vi "输入数据解析.vi"(0 "单个参数补充":dbl, 1 "从板号":dbl=1.0, 2 "主板二维码":string="BNET01", 3 "从板二维码":string="BNET01", 5 "主板引用":refnum<vi>, 7 "从板引用":refnum<vi>, 9 "主板选项":string="三级故障阀值", 11 "枚举":enum16{"主板", "从板"}(ring), 12 "快换":bool caption="快换写入") -> (4 "输出数组":dbl[][](array[numeric]), 6 "数组长度":dbl[](array[numeric]), 8 "循环次数":i32, 10 "命令":u32, 14 "名称":string[](array[string]), 15 "命令序号":u32[](array[numeric]))   [LabVIEW 2013] (continued)
              tunnel: [w18491 w18502 w18513 w18524 w18534 w18544 w18555] -> w18485
              frame 0, Default {
                # "电压过高"
                n7255 = disable-structure shown="启用" {
                  disable-tunnel: [w18497 w18500] -> w18493
                  disable-tunnel: [w18496 w18500] -> w18492
                  disable-tunnel: w18490 -> [w18495 _]
                  frame Disabled {
                    n7256 = Unbundle By Name(w18495) -> ("电压过高"=w18494:dbl)
                    n7257 = call "输入分辨率计算-EV05.vi"("1字节?"=FALSE, "数值"=w18494, "分辨率"=0.1) -> ("低字节"=w18496:dbl, "高字节1"=w18497:dbl)  [unwired: 2 in, 5 out]
                  }
                  frame Enabled {
                    w18500 = 255 ("高字节1")
                  }
                }
                n7258 = Build Array(w18493, w18492) -> (w18491:i32[])
              }
              frame 1 {
                # "电压过低"
                n7259 = disable-structure shown="启用" {
                  disable-tunnel: [w18508 w18511] -> w18504
                  disable-tunnel: [w18507 w18511] -> w18503
                  disable-tunnel: w18501 -> [w18506 _]
                  frame Disabled {
                    n7260 = Unbundle By Name(w18506) -> ("电压过低"=w18505:dbl)
                    n7261 = call "输入分辨率计算-EV05.vi"("1字节?"=FALSE, "数值"=w18505, "分辨率"=0.1) -> ("低字节"=w18507:dbl, "高字节1"=w18508:dbl)  [unwired: 2 in, 5 out]
                  }
                  frame Enabled {
                    w18511 = 255 ("高字节1")
                  }
                }
                n7262 = Build Array(w18504, w18503) -> (w18502:i32[])
              }
              frame 2 {
                # "电压不均衡"
                n7263 = disable-structure shown="启用" {
                  disable-tunnel: [w18519 w18522] -> w18515
                  disable-tunnel: [w18518 w18522] -> w18514
                  disable-tunnel: w18512 -> [w18517 _]
                  frame Disabled {
                    n7264 = Unbundle By Name(w18517) -> ("电压不均衡(V)"=w18516:dbl)
                    n7265 = call "输入分辨率计算-EV05.vi"("1字节?"=FALSE, "数值"=w18516, "分辨率"=0.1) -> ("低字节"=w18518:dbl, "高字节1"=w18519:dbl)  [unwired: 2 in, 5 out]
                  }
                  frame Enabled {
                    w18522 = 255 ("高字节1")
                  }
                }
                n7266 = Build Array(w18515, w18514) -> (w18513:i32[])
              }
              frame 3 {
                # "温度过高"
                n7267 = disable-structure shown="启用" {
                  disable-tunnel: [w18529 255 ("高字节1")] -> w18525
                  disable-tunnel: w18523 -> [w18527 _]
                  frame Disabled {
                    n7268 = Unbundle By Name(w18527) -> ("温度过高"=w18526:dbl)
                    n7269 = call "输入分辨率计算-EV05.vi"("1字节?"=TRUE, "数值"=w18526, "偏移量"=-40.0, "分辨率"=1.0) -> ("高字节1"=w18529:dbl)  [unwired: 1 in, 6 out]
                  }
                  frame Enabled {
                  }
                }
                n7270 = Build Array(w18525) -> (w18524:i32[])
              }
              frame 4 {
                # "温度过低"
                n7271 = disable-structure shown="启用" {
                  disable-tunnel: [w18539 255 ("高字节1")] -> w18535
                  disable-tunnel: w18533 -> [w18537 _]
                  frame Disabled {
                    n7272 = Unbundle By Name(w18537) -> ("温度过低"=w18536:dbl)
                    n7273 = call "输入分辨率计算-EV05.vi"("1字节?"=TRUE, "数值"=w18536, "偏移量"=-40.0, "分辨率"=1.0) -> ("高字节1"=w18539:dbl)  [unwired: 1 in, 6 out]
                  }
                  frame Enabled {
                  }
                }
                n7274 = Build Array(w18535) -> (w18534:i32[])
              }
              frame 5 {
                # "温度不均衡"
                n7275 = disable-structure shown="启用" {
                  disable-tunnel: [w18548 255 ("高字节1")] -> w18545
                  disable-tunnel: w18543 -> [w18547 _]
                  frame Disabled {
                    n7276 = Unbundle By Name(w18547) -> ("温度不均衡"=w18546:dbl)
                    n7277 = call "输入分辨率计算-EV05.vi"("1字节?"=TRUE, "数值"=w18546, "分辨率"=1.0) -> ("高字节1"=w18548:dbl)  [unwired: 2 in, 6 out]
                  }
                  frame Enabled {
                  }
                }
                n7278 = Build Array(w18545) -> (w18544:i32[])
              }
              frame 6 {
                # "SOC过低"
                n7279 = disable-structure shown="启用" {
                  disable-tunnel: w18554 -> [w18559 _]
                  disable-tunnel: [w18556 w18562] -> w18553
                  disable-tunnel: [w18557 w18562] -> w18552
                  frame Enabled {
                    n7280 = Unbundle By Name(w18559) -> ("SOC过低"=w18558:dbl)
                    n7281 = call "输入分辨率计算-EV05.vi"("1字节?"=FALSE, "数值"=w18558, "分辨率"=0.1) -> ("低字节"=w18556:dbl, "高字节1"=w18557:dbl)  [unwired: 2 in, 5 out]
                  }
                  frame Disabled {
                    w18562 = 255 ("高字节1")
                  }
                }
                n7282 = Build Array(w18552, w18553) -> (w18555:dbl[])
              }
            }
            n7283 = Insert Into Array(array=w18486, new element=w18485) -> (w18487:dbl[])  [unwired: 1 in]
          }
          n7284 = Build Array(w18480) -> (w18479:dbl[][])
        }
        frame "SOC过低(2)" {
          n7285 = Unbundle By Name(w18567) -> ("二级故障(从板)"=w18568:refnum<vi>)
          n7286 = property class="Clust (严格)"(reference=w18568) -> ("Value"=w18566:T8)  [unwired: 1 in, 2 out]
          n7287 = for {
            N: 7 -> [_]
            tunnel: w18566 -> [w18578]
            shift-right: [w18577] -> w18570
            shift-left: dbl[] [] -> [w18576]
            i -> [w18579]
            n7288 = case shown="6" w18579 {
              tunnel: w18578 -> [w18580 w18591 w18602 w18613 w18623 w18633 w18644]
              tunnel: [w18581 w18592 w18603 w18614 w18624 w18634 w18645] -> w18575
              frame 0, Default {
                # "电压过高"
                n7289 = disable-structure shown="启用" {
                  disable-tunnel: [w18587 w18590] -> w18583
                  disable-tunnel: [w18586 w18590] -> w18582
                  disable-tunnel: w18580 -> [w18585 _]
                  frame Disabled {
                    n7290 = Unbundle By Name(w18585) -> ("电压过高"=w18584:dbl)
                    n7291 = call "输入分辨率计算-EV05.vi"("1字节?"=FALSE, "数值"=w18584, "分辨率"=0.1) -> ("低字节"=w18586:dbl, "高字节1"=w18587:dbl)  [unwired: 2 in, 5 out]
                  }
                  frame Enabled {
                    w18590 = 255 ("高字节1")
                  }
                }
                n7292 = Build Array(w18583, w18582) -> (w18581:i32[])
              }
              frame 1 {
                # "电压过低"
                n7293 = disable-structure shown="启用" {
                  disable-tunnel: [w18598 w18601] -> w18594
                  disable-tunnel: [w18597 w18601] -> w18593
                  disable-tunnel: w18591 -> [w18596 _]
                  frame Disabled {
                    n7294 = Unbundle By Name(w18596) -> ("电压过低"=w18595:dbl)
                    n7295 = call "输入分辨率计算-EV05.vi"("1字节?"=FALSE, "数值"=w18595, "分辨率"=0.1) -> ("低字节"=w18597:dbl, "高字节1"=w18598:dbl)  [unwired: 2 in, 5 out]
                  }
                  frame Enabled {
                    w18601 = 255 ("高字节1")
                  }
                }
                n7296 = Build Array(w18594, w18593) -> (w18592:i32[])
              }
              frame 2 {
                # "电压不均衡"
                n7297 = disable-structure shown="启用" {
                  disable-tunnel: [w18609 w18612] -> w18605
                  disable-tunnel: [w18608 w18612] -> w18604
                  disable-tunnel: w18602 -> [w18607 _]
                  frame Disabled {
                    n7298 = Unbundle By Name(w18607) -> ("电压不均衡(V)"=w18606:dbl)
                    n7299 = call "输入分辨率计算-EV05.vi"("1字节?"=FALSE, "数值"=w18606, "分辨率"=0.1) -> ("低字节"=w18608:dbl, "高字节1"=w18609:dbl)  [unwired: 2 in, 5 out]
                  }
                  frame Enabled {
                    w18612 = 255 ("高字节1")
                  }
                }
                n7300 = Build Array(w18605, w18604) -> (w18603:i32[])
              }
              frame 3 {
                # "温度过高"
                n7301 = disable-structure shown="启用" {
                  disable-tunnel: [w18619 255 ("高字节1")] -> w18615
                  disable-tunnel: w18613 -> [w18617 _]
                  frame Disabled {
                    n7302 = Unbundle By Name(w18617) -> ("温度过高"=w18616:dbl)
                    n7303 = call "输入分辨率计算-EV05.vi"("1字节?"=TRUE, "数值"=w18616, "偏移量"=-40.0, "分辨率"=1.0) -> ("高字节1"=w18619:dbl)  [unwired: 1 in, 6 out]
                  }
                  frame Enabled {
                  }
                }
                n7304 = Build Array(w18615) -> (w18614:i32[])
              }
              frame 4 {
                # "温度过低"
                n7305 = disable-structure shown="启用" {
                  disable-tunnel: [w18629 255 ("高字节1")] -> w18625
                  disable-tunnel: w18623 -> [w18627 _]
                  frame Disabled {
                    n7306 = Unbundle By Name(w18627) -> ("温度过低"=w18626:dbl)
                    n7307 = call "输入分辨率计算-EV05.vi"("1字节?"=TRUE, "数值"=w18626, "偏移量"=-40.0, "分辨率"=1.0) -> ("高字节1"=w18629:dbl)  [unwired: 1 in, 6 out]
                  }
                  frame Enabled {
                  }
                }
                n7308 = Build Array(w18625) -> (w18624:i32[])
              }
              frame 5 {
                # "温度不均衡"
                n7309 = disable-structure shown="启用" {
                  disable-tunnel: [w18638 255 ("高字节1")] -> w18635
                  disable-tunnel: w18633 -> [w18637 _]
                  frame Disabled {
                    n7310 = Unbundle By Name(w18637) -> ("温度不均衡"=w18636:dbl)
                    n7311 = call "输入分辨率计算-EV05.vi"("1字节?"=TRUE, "数值"=w18636, "分辨率"=1.0) -> ("高字节1"=w18638:dbl)  [unwired: 2 in, 6 out]
                  }
                  frame Enabled {
                  }
                }
                n7312 = Build Array(w18635) -> (w18634:i32[])
              }
              frame 6 {
                # "SOC过低"
                n7313 = disable-structure shown="启用" {
                  disable-tunnel: w18644 -> [w18649 _]
                  disable-tunnel: [w18646 w18652] -> w18643
                  disable-tunnel: [w18647 w18652] -> w18642
                  frame Enabled {
                    n7314 = Unbundle By Name(w18649) -> ("SOC过低"=w18648:dbl)
                    n7315 = call "输入分辨率计算-EV05.vi"("1字节?"=FALSE, "数值"=w18648, "分辨率"=0.1) -> ("低字节"=w18646:dbl, "高字节1"=w18647:dbl)  [unwired: 2 in, 5 out]
                  }
                  frame Disabled {
                    w18652 = 255 ("高字节1")
                  }
                }
                n7316 = Build Array(w18642, w18643) -> (w18645:dbl[])
              }
            }
            n7317 = Insert Into Array(array=w18576, new element=w18575) -> (w18577:dbl[])  [unwired: 1 in]
          }
          n7318 = Build Array(w18570) -> (w18569:dbl[][])
        }
        frame "SOC过低(3)" {
          n7319 = Unbundle By Name(w18657) -> ("三级故障(从板)"=w18658:refnum<vi>)
          n7320 = property class="Clust (严格)"(reference=w18658) -> ("Value"=w18656:T8)  [unwired: 1 in, 2 out]
          n7321 = for {
            N: 7 -> [_]
            tunnel: w18656 -> [w18668]
            shift-right: [w18667] -> w18660
            shift-left: dbl[] [] -> [w18666]
            i -> [w18669]
            n7322 = case shown="6" w18669 {
              tunnel: w18668 -> [w18670 w18681 w18692 w18703 w18713 w18723 w18734]
              tunnel: [w18671 w18682 w18693 w18704 w18714 w18724 w18735] -> w18665
              frame 0, Default {
                # "电压过高"
                n7323 = disable-structure shown="启用" {
                  disable-tunnel: [w18677 w18680] -> w18673
                  disable-tunnel: [w18676 w18680] -> w18672
                  disable-tunnel: w18670 -> [w18675 _]
                  frame Disabled {
                    n7324 = Unbundle By Name(w18675) -> ("电压过高"=w18674:dbl)
                    n7325 = call "输入分辨率计算-EV05.vi"("1字节?"=FALSE, "数值"=w18674, "分辨率"=0.1) -> ("低字节"=w18676:dbl, "高字节1"=w18677:dbl)  [unwired: 2 in, 5 out]
                  }
                  frame Enabled {
                    w18680 = 255 ("高字节1")
                  }
                }
                n7326 = Build Array(w18673, w18672) -> (w18671:i32[])
              }
              frame 1 {
                # "电压过低"
                n7327 = disable-structure shown="启用" {
                  disable-tunnel: [w18688 w18691] -> w18684
                  disable-tunnel: [w18687 w18691] -> w18683
                  disable-tunnel: w18681 -> [w18686 _]
                  frame Disabled {
                    n7328 = Unbundle By Name(w18686) -> ("电压过低"=w18685:dbl)
                    n7329 = call "输入分辨率计算-EV05.vi"("1字节?"=FALSE, "数值"=w18685, "分辨率"=0.1) -> ("低字节"=w18687:dbl, "高字节1"=w18688:dbl)  [unwired: 2 in, 5 out]
                  }
                  frame Enabled {
                    w18691 = 255 ("高字节1")
                  }
                }
                n7330 = Build Array(w18684, w18683) -> (w18682:i32[])
              }
              frame 2 {
                # "电压不均衡"
                n7331 = disable-structure shown="启用" {
                  disable-tunnel: [w18699 w18702] -> w18695
                  disable-tunnel: [w18698 w18702] -> w18694
                  disable-tunnel: w18692 -> [w18697 _]
                  frame Disabled {
                    n7332 = Unbundle By Name(w18697) -> ("电压不均衡(V)"=w18696:dbl)
                    n7333 = call "输入分辨率计算-EV05.vi"("1字节?"=FALSE, "数值"=w18696, "分辨率"=0.1) -> ("低字节"=w18698:dbl, "高字节1"=w18699:dbl)  [unwired: 2 in, 5 out]
                  }
                  frame Enabled {
                    w18702 = 255 ("高字节1")
                  }
                }
                n7334 = Build Array(w18695, w18694) -> (w18693:i32[])
              }
              frame 3 {
                # "温度过高"
                n7335 = disable-structure shown="启用" {
                  disable-tunnel: [w18709 255 ("高字节1")] -> w18705
                  disable-tunnel: w18703 -> [w18707 _]
                  frame Disabled {
                    n7336 = Unbundle By Name(w18707) -> ("温度过高"=w18706:dbl)
                    n7337 = call "输入分辨率计算-EV05.vi"("1字节?"=TRUE, "数值"=w18706, "偏移量"=-40.0, "分辨率"=1.0) -> ("高字节1"=w18709:dbl)  [unwired: 1 in, 6 out]
                  }
                  frame Enabled {
                  }
                }
                n7338 = Build Array(w18705) -> (w18704:i32[])
              }
              frame 4 {
                # "温度过低"
                n7339 = disable-structure shown="启用" {
                  disable-tunnel: [w18719 255 ("高字节1")] -> w18715
                  disable-tunnel: w18713 -> [w18717 _]
                  frame Disabled {
                    n7340 = Unbundle By Name(w18717) -> ("温度过低"=w18716:dbl)
                    n7341 = call "输入分辨率计算-EV05.vi"("1字节?"=TRUE, "数值"=w18716, "偏移量"=-40.0, "分辨率"=1.0) -> ("高字节1"=w18719:dbl)  [unwired: 1 in, 6 out]
                  }
                  frame Enabled {
                  }
                }
                n7342 = Build Array(w18715) -> (w18714:i32[])
              }
              frame 5 {
                # "温度不均衡"
                n7343 = disable-structure shown="启用" {
                  disable-tunnel: [w18728 255 ("高字节1")] -> w18725
                  disable-tunnel: w18723 -> [w18727 _]
                  frame Disabled {
                    n7344 = Unbundle By Name(w18727) -> ("温度不均衡"=w18726:dbl)
                    n7345 = call "输入分辨率计算-EV05.vi"("1字节?"=TRUE, "数值"=w18726, "分辨率"=1.0) -> ("高字节1"=w18728:dbl)  [unwired: 2 in, 6 out]
                  }
                  frame Enabled {
                  }
                }
                n7346 = Build Array(w18725) -> (w18724:i32[])
              }
              frame 6 {
                # "SOC过低"
                n7347 = disable-structure shown="启用" {
                  disable-tunnel: w18734 -> [w18739 _]
                  disable-tunnel: [w18736 w18742] -> w18733
                  disable-tunnel: [w18737 w18742] -> w18732
                  frame Enabled {
                    n7348 = Unbundle By Name(w18739) -> ("SOC过低"=w18738:dbl)
                    n7349 = call "输入分辨率计算-EV05.vi"("1字节?"=FALSE, "数值"=w18738, "分辨率"=0.1) -> ("低字节"=w18736:dbl, "高字节1"=w18737:dbl)  [unwired: 2 in, 5 out]
                  }
                  frame Disabled {
                    w18742 = 255 ("高字节1")
                  }
                }
                n7350 = Build Array(w18732, w18733) -> (w18735:dbl[])
              }
            }
            n7351 = Insert Into Array(array=w18666, new element=w18665) -> (w18667:dbl[])  [unwired: 1 in]
          }
          n7352 = Build Array(w18660) -> (w18659:dbl[][])
        }
        frame "二级故障阀值" {
          n7353 = Unbundle By Name(w18747) -> ("二级故障(从板)"=w18748:refnum<vi>)
          n7354 = property class="Clust (严格)"(reference=w18748) -> ("Value"=w18746:T8)  [unwired: 1 in, 2 out]
          n7355 = for {
            N: 7 -> [_]
            tunnel: w18746 -> [w18758]
            shift-right: [w18757] -> w18750
            shift-left: dbl[] [] -> [w18756]
            i -> [w18759]
            n7356 = case shown="5" w18759 {
              tunnel: w18758 -> [w18761 w18768 w18775 w18782 w18789 w18796 w18804]
              tunnel: [w18762 w18769 w18776 w18784 w18791 w18797 w18805] -> w18755
              frame 0, Default {
                # "电压过高"
                n7357 = Unbundle By Name(w18761) -> ("电压过高"=w18760:dbl)
                n7358 = call "输入分辨率计算-EV05.vi"("1字节?"=FALSE, "数值"=w18760, "分辨率"=0.001) -> ("低字节"=w18763:dbl, "高字节1"=w18764:dbl)  [unwired: 2 in, 5 out]
                n7359 = Build Array(w18764, w18763) -> (w18762:dbl[])
              }
              frame 1 {
                # "电压过低"
                n7360 = Unbundle By Name(w18768) -> ("电压过低"=w18767:dbl)
                n7361 = call "输入分辨率计算-EV05.vi"("1字节?"=FALSE, "数值"=w18767, "分辨率"=0.001) -> ("低字节"=w18770:dbl, "高字节1"=w18771:dbl)  [unwired: 2 in, 5 out]
                n7362 = Build Array(w18771, w18770) -> (w18769:dbl[])
              }
              frame 2 {
                # "电压不均衡"
                n7363 = Unbundle By Name(w18775) -> ("电压不均衡(V)"=w18774:dbl)
                n7364 = call "输入分辨率计算-EV05.vi"("1字节?"=FALSE, "数值"=w18774, "分辨率"=0.001) -> ("低字节"=w18777:dbl, "高字节1"=w18778:dbl)  [unwired: 2 in, 5 out]
                n7365 = Build Array(w18778, w18777) -> (w18776:dbl[])
              }
              frame 3 {
                # "温度不均衡"
                n7366 = Unbundle By Name(w18782) -> ("温度过高"=w18781:dbl)
                n7367 = call "输入分辨率计算-EV05.vi"("1字节?"=TRUE, "数值"=w18781, "偏移量"=-40.0, "分辨率"=1.0) -> ("高字节1"=w18785:dbl)  [unwired: 1 in, 6 out]
                n7368 = Build Array(w18785) -> (w18784:dbl[])
              }
              frame 4 {
                # "温度过低"
                n7369 = Unbundle By Name(w18789) -> ("温度过低"=w18788:dbl)
                n7370 = call "输入分辨率计算-EV05.vi"("1字节?"=TRUE, "数值"=w18788, "偏移量"=-40.0, "分辨率"=1.0) -> ("高字节1"=w18792:dbl)  [unwired: 1 in, 6 out]
                n7371 = Build Array(w18792) -> (w18791:dbl[])
              }
              frame 5 {
                # "温度不均衡"
                n7372 = Unbundle By Name(w18796) -> ("温度不均衡"=w18795:dbl)
                n7373 = call "输入分辨率计算-EV05.vi"("1字节?"=TRUE, "数值"=w18795, "分辨率"=1.0) -> ("高字节1"=w18798:dbl)  [unwired: 2 in, 6 out]
                n7374 = Build Array(w18798) -> (w18797:dbl[])
              }
              frame 6 {
                # "SOC过低"
                n7375 = Unbundle By Name(w18804) -> ("SOC过低"=w18803:dbl)
                n7376 = call "输入分辨率计算-EV05.vi"("1字节?"=FALSE, "数值"=w18803, "分辨率"=0.1) -> ("低字节"=w18801:dbl, "高字节1"=w18802:dbl)  [unwired: 2 in, 5 out]
                n7377 = Build Array(w18802, w18801) -> (w18805:dbl[])
              }
            }
            n7378 = Insert Into Array(array=w18756, new element=w18755) -> (w18757:dbl[])  [unwired: 1 in]
          }
          n7379 = Build Array(w18750) -> (w18749:dbl[][])
        }
        frame "三级故障阀值" {
          n7380 = Unbundle By Name(w18812) -> ("三级故障(从板)"=w18813:refnum<vi>)
          n7381 = property class="Clust (严格)"(reference=w18813) -> ("Value"=w18811:T8)  [unwired: 1 in, 2 out]
          n7382 = for {
            N: 7 -> [_]
            tunnel: w18811 -> [w18823]
            shift-right: [w18822] -> w18815
            shift-left: dbl[] [] -> [w18821]
            i -> [w18824]
            n7383 = case shown="2" w18824 {
              tunnel: w18823 -> [w18826 w18833 w18840 w18847 w18854 w18861 w18869]
              tunnel: [w18827 w18834 w18841 w18849 w18856 w18862 w18870] -> w18820
              frame 0, Default {
                # "电压过高"
                n7384 = Unbundle By Name(w18826) -> ("电压过高"=w18825:dbl)
                n7385 = call "输入分辨率计算-EV05.vi"("1字节?"=FALSE, "数值"=w18825, "分辨率"=0.001) -> ("低字节"=w18828:dbl, "高字节1"=w18829:dbl)  [unwired: 2 in, 5 out]
                n7386 = Build Array(w18829, w18828) -> (w18827:dbl[])
              }
              frame 1 {
                # "电压过低"
                n7387 = Unbundle By Name(w18833) -> ("电压过低"=w18832:dbl)
                n7388 = call "输入分辨率计算-EV05.vi"("1字节?"=FALSE, "数值"=w18832, "分辨率"=0.001) -> ("低字节"=w18835:dbl, "高字节1"=w18836:dbl)  [unwired: 2 in, 5 out]
                n7389 = Build Array(w18836, w18835) -> (w18834:dbl[])
              }
              frame 2 {
                # "电压不均衡"
                n7390 = Unbundle By Name(w18840) -> ("电压不均衡(V)"=w18839:dbl)
                n7391 = call "输入分辨率计算-EV05.vi"("1字节?"=FALSE, "数值"=w18839, "分辨率"=0.001) -> ("低字节"=w18842:dbl, "高字节1"=w18843:dbl)  [unwired: 2 in, 5 out]
                n7392 = Build Array(w18843, w18842) -> (w18841:dbl[])
              }
              frame 3 {
                # "温度不均衡"
                n7393 = Unbundle By Name(w18847) -> ("温度过高"=w18846:dbl)
                n7394 = call "输入分辨率计算-EV05.vi"("1字节?"=TRUE, "数值"=w18846, "偏移量"=-40.0, "分辨率"=1.0) -> ("高字节1"=w18850:dbl)  [unwired: 1 in, 6 out]
                n7395 = Build Array(w18850) -> (w18849:dbl[])
              }
              frame 4 {
                # "温度过低"
                n7396 = Unbundle By Name(w18854) -> ("温度过低"=w18853:dbl)
                n7397 = call "输入分辨率计算-EV05.vi"("1字节?"=TRUE, "数值"=w18853, "偏移量"=-40.0, "分辨率"=1.0) -> ("高字节1"=w18857:dbl)  [unwired: 1 in, 6 out]
                n7398 = Build Array(w18857) -> (w18856:dbl[])
              }
              frame 5 {
                # "温度不均衡"
                n7399 = Unbundle By Name(w18861) -> ("温度不均衡"=w18860:dbl)
                n7400 = call "输入分辨率计算-EV05.vi"("1字节?"=TRUE, "数值"=w18860, "分辨率"=1.0) -> ("高字节1"=w18863:dbl)  [unwired: 2 in, 6 out]
                n7401 = Build Array(w18863) -> (w18862:dbl[])
              }
              frame 6 {
                # "SOC过低"
                n7402 = Unbundle By Name(w18869) -> ("SOC过低"=w18868:dbl)
                n7403 = call "输入分辨率计算-EV05.vi"("1字节?"=FALSE, "数值"=w18868, "分辨率"=0.1) -> ("低字节"=w18866:dbl, "高字节1"=w18867:dbl)  [unwired: 2 in, 5 out]
                n7404 = Build Array(w18867, w18866) -> (w18870:dbl[])
              }
            }
            n7405 = Insert Into Array(array=w18821, new element=w18820) -> (w18822:dbl[])  [unwired: 1 in]
          }
          n7406 = Build Array(w18815) -> (w18814:dbl[][])
        }
        frame "快换参数" {
          n7407 = case shown="真" w18876 {
            tunnel: [_ w18889] -> w18880
            tunnel: [_ w18888] -> w18879
            tunnel: w18878 -> [_ w18884]
            tunnel: [_ w18887] -> w18877
            tunnel: [_ u32 35 ("命令序号")] -> w18875
            tunnel: [_ w18882] -> w18874
            tunnel: [_ w18881] -> w18873
            frame False {
            }
            frame True {
              w18882 = 7
              n7408 = Unbundle By Name(w18884) -> ("电池组信息(从板)"=w18885:refnum<vi>)
              n7409 = property class="Clust (严格)"(reference=w18885) -> ("Value"=w18883:T9)  [unwired: 1 in, 2 out]
              n7410 = for {
                N: w18882 -> [_]
                tunnel: [w18895] -> w18889 mode=indexing
                tunnel: [w18894] -> w18888 mode=indexing
                tunnel: w18883 -> [w18893]
                tunnel: [w18892] -> w18887 mode=indexing
                tunnel: [w18890] -> w18881 mode=indexing
                i -> [w18891]
                n7411 = case shown="3" w18891 {
                  tunnel: [30 ("单个参数补充") 4 ("单个参数补充") 8 ("单个参数补充") 6 ("单个参数补充") 4 ("单个参数补充") 8 ("单个参数补充") 14 ("单个参数补充")] -> w18895
                  tunnel: [u32 1 ("命令序号") u32 2 ("命令序号") u32 3 ("命令序号") u32 4 ("命令序号") u32 5 ("命令序号") u32 6 ("命令序号") u32 7 ("命令序号")] -> w18894
                  tunnel: w18893 -> [w18899 w18974 w18982 w19012 w19023 w19031 w19052]
                  tunnel: [w18896 w18967 w18999 w19014 w19024 w19029 w19054] -> w18892
                  tunnel: ["电池包信息1" "电池包序号" "充放电安时" "充电次数时间" "SOC" "车牌号" "充电参数"] -> w18890
                  frame 0, Default {
                    w18909 = ":" ("正则表达式")
                    w18917 = 0.0 ("元素")
                    w18936 = 256.0 ("y")
                    w18941 = 256.0 ("y")
                    w18954 = 2 ("偏移量(0)")
                    w18951 = "-" ("正则表达式")
                    # "电池组信息"
                    n7412 = Unbundle By Name(w18899) -> ("串联数"=w18958:dbl, "并联数"=w18957:dbl, "电池厂家"=w18897:dbl, "电池类型"=w18898:dbl, "生产日期"=w18956:string)
                    n7413 = Unbundle By Name(w18899) -> ("额定能量"=w18922:dbl, "额定容量"=w18924:dbl, "实际容量"=w18923:dbl, "额定总压"=w18947:dbl)
                    n7414 = Match Pattern(string=w18956, regular expression=w18951) -> (before substring=w18955:string, after substring=w18952:string)  [unwired: 3 out]
                    n7415 = Match Pattern(string=w18952, regular expression=w18951) -> (before substring=w18950:string, after substring=w18915:string)  [unwired: 3 out]
                    n7416 = Match Pattern(string=w18915, regular expression=" " ("正则表达式")) -> (before substring=w18913:string, after substring=w18912:string)  [unwired: 3 out]
                    n7417 = call "输入分辨率计算-EV05.vi"("1字节?"=FALSE, "数值"=w18922, "分辨率"=0.1) -> ("低字节"=w18921:dbl, "高字节1"=w18920:dbl)  [unwired: 2 in, 5 out]
                    n7418 = String Subset(string=w18955, offset (0)=w18954, length (rest)=w18954) -> (substring=w18953:string)
                    n7419 = call "输入分辨率计算-EV05.vi"("1字节?"=TRUE, "数值 2"=w18923, "数值"=w18924, "分辨率"=0.001) -> ("高字节 2"=w18925:dbl, "高字节1"=w18926:dbl)  [unwired: 1 in, 5 out]
                    n7420 = Match Pattern(string=w18912, regular expression=w18909) -> (before substring=w18911:string, after substring=w18910:string)  [unwired: 3 out]
                    n7421 = Fract/Exp String To Number(string=w18953) -> (number=w18905:dbl)  [unwired: 1 in, 3 out]
                    n7422 = Fract/Exp String To Number(string=w18950) -> (number=w18904:dbl)  [unwired: 4 out]
                    n7423 = Fract/Exp String To Number(string=w18913) -> (number=w18903:dbl)  [unwired: 4 out]
                    n7424 = Match Pattern(string=w18910, regular expression=w18909) -> (before substring=w18908:string, after substring=w18907:string)  [unwired: 3 out]
                    n7425 = call "输入分辨率计算-EV05.vi"("1字节?"=FALSE, "数值"=w18947, "分辨率"=0.1) -> ("低字节"=w18918:dbl, "高字节1"=w18919:dbl)  [unwired: 2 in, 5 out]
                    n7426 = Quotient & Remainder(x=w18926, y=w18941) -> (x-y*floor(x/y)=w18940:dbl, floor(x/y)=w18944:dbl)
                    n7427 = Fract/Exp String To Number(string=w18911) -> (number=w18902:dbl)  [unwired: 4 out]
                    n7428 = Quotient & Remainder(x=w18925, y=w18936) -> (x-y*floor(x/y)=w18932:dbl, floor(x/y)=w18933:dbl)
                    n7429 = Quotient & Remainder(x=w18944, y=w18941) -> (x-y*floor(x/y)=w18939:dbl, floor(x/y)=w18943:dbl)
                    n7430 = Fract/Exp String To Number(string=w18908) -> (number=w18901:dbl)  [unwired: 4 out]
                    n7431 = Quotient & Remainder(x=w18933, y=w18936) -> (x-y*floor(x/y)=w18931:dbl, floor(x/y)=w18934:dbl)
                    n7432 = call <vilib>:"Trim Whitespace.vi"("string"=w18907) -> ("trimmed string"=w18906:string)  [unwired: 1 in]
                    n7433 = Quotient & Remainder(x=w18943, y=w18941) -> (x-y*floor(x/y)=w18938:dbl, floor(x/y)=w18942:dbl)
                    n7434 = Quotient & Remainder(x=w18934, y=w18936) -> (x-y*floor(x/y)=w18930:dbl, floor(x/y)=w18935:dbl)
                    n7435 = Quotient & Remainder(x=w18958, y=256.0) -> (x-y*floor(x/y)=w18960:dbl, floor(x/y)=w18961:dbl)
                    n7436 = Fract/Exp String To Number(string=w18906) -> (number=w18900:dbl)  [unwired: 4 out]
                    n7437 = Quotient & Remainder(x=w18942, y=w18941) -> (x-y*floor(x/y)=w18937:dbl)  [unwired: 1 out]
                    n7438 = Quotient & Remainder(x=w18935, y=w18936) -> (x-y*floor(x/y)=w18929:dbl)  [unwired: 1 out]
                    n7439 = Build Array(w18920, w18921, w18937, w18938, w18939, w18940, w18929, w18930, w18931, w18932, w18919, w18918, w18917, w18917, w18917, w18905, w18904, w18903, w18902, w18901, w18900) -> (w18916:dbl[])
                    n7440 = Build Array(w18961, w18960, w18957, w18897, w18898) -> (w18959:dbl[])
                    n7441 = Insert Into Array(array=w18959, new element=w18916) -> (w18896:dbl[])  [unwired: 1 in]
                  }
                  frame 1 {
                    n7442 = Unbundle By Name(w18974) -> ("电池包序号"=w18971:dbl)
                    n7443 = Quotient & Remainder(x=w18971, y=256.0) -> (x-y*floor(x/y)=w18968:dbl, floor(x/y)=w18969:dbl)
                    n7444 = Build Array(w18969, w18968) -> (w18967:dbl[])
                  }
                  frame 2 {
                    w18990 = 256.0 ("y")
                    w18995 = 256.0 ("y")
                    # "充放电安时/安时数"
                    n7445 = Unbundle By Name(w18982) -> ("充电总安时"=w18979:dbl, "放电总这时"=w18978:dbl)
                    n7446 = call "输入分辨率计算-EV05.vi"("1字节?"=TRUE, "数值 2"=w18978, "数值"=w18979, "分辨率"=0.001) -> ("高字节 2"=w18976:dbl, "高字节1"=w18977:dbl)  [unwired: 1 in, 5 out]
                    n7447 = Quotient & Remainder(x=w18977, y=w18995) -> (x-y*floor(x/y)=w18994:dbl, floor(x/y)=w18998:dbl)
                    n7448 = Quotient & Remainder(x=w18976, y=w18990) -> (x-y*floor(x/y)=w18986:dbl, floor(x/y)=w18987:dbl)
                    n7449 = Quotient & Remainder(x=w18998, y=w18995) -> (x-y*floor(x/y)=w18993:dbl, floor(x/y)=w18997:dbl)
                    n7450 = Quotient & Remainder(x=w18987, y=w18990) -> (x-y*floor(x/y)=w18985:dbl, floor(x/y)=w18988:dbl)
                    n7451 = Quotient & Remainder(x=w18997, y=w18995) -> (x-y*floor(x/y)=w18992:dbl, floor(x/y)=w18996:dbl)
                    n7452 = Quotient & Remainder(x=w18988, y=w18990) -> (x-y*floor(x/y)=w18984:dbl, floor(x/y)=w18989:dbl)
                    n7453 = Quotient & Remainder(x=w18996, y=w18995) -> (x-y*floor(x/y)=w18991:dbl)  [unwired: 1 out]
                    n7454 = Quotient & Remainder(x=w18989, y=w18990) -> (x-y*floor(x/y)=w18983:dbl)  [unwired: 1 out]
                    n7455 = Build Array(w18991, w18992, w18993, w18994, w18983, w18984, w18985, w18986) -> (w18999:dbl[])
                  }
                  frame 3 {
                    w19007 = 256.0 ("y")
                    # "充电次数"
                    n7456 = Unbundle By Name(w19012) -> ("放空次数"=w19011:dbl, "充满次数"=w19009:dbl, "充电次数"=w19008:dbl)
                    n7457 = Quotient & Remainder(x=w19011, y=w19007) -> (x-y*floor(x/y)=w19013:dbl, floor(x/y)=w19010:dbl)
                    n7458 = Quotient & Remainder(x=w19009, y=w19007) -> (x-y*floor(x/y)=w19005:dbl, floor(x/y)=w19006:dbl)
                    n7459 = Quotient & Remainder(x=w19008, y=w19007) -> (x-y*floor(x/y)=w19003:dbl, floor(x/y)=w19004:dbl)
                    n7460 = Build Array(w19010, w19013, w19006, w19005, w19004, w19003) -> (w19014:dbl[])
                  }
                  frame 4 {
                    # "SOC"
                    n7461 = Unbundle By Name(w19023) -> ("SOC"=w19022:dbl)
                    n7462 = call "输入分辨率计算-EV05.vi"("1字节?"=FALSE, "数值"=w19022, "分辨率"=0.1) -> ("低字节"=w19018:dbl, "高字节1"=w19019:dbl)  [unwired: 2 in, 5 out]
                    n7463 = Build Array(w19019, w19018) -> (w19024:dbl[])
                  }
                  frame 5 {
                    # "车牌号"
                    n7464 = Unbundle By Name(w19031) -> ("车牌号"=w19030:string)
                    n7465 = String To Byte Array(string=w19030) -> (unsigned byte array=w19034:u8[])
                    n7466 = Array Subset(array=w19034, length=8 ("长度")) -> (w19029:u8[])  [unwired: 1 in]
                  }
                  frame 6 {
                    n7467 = Unbundle By Name(w19052) -> ("最大允许单体电压"=w19050:dbl, "最大允许总电压"=w19049:dbl, "最大允许温度"=w19048:dbl, "最小允许温度"=w19047:dbl, "最大允许充电电流"=w19046:dbl, "最小允许充电电流"=w19045:dbl, "电流步长"=w19041:dbl, "最小允许单体电压"=w19044:dbl)
                    n7468 = call "输入分辨率计算-EV05.vi"("1字节?"=FALSE, "数值 2"=w19044, "数值"=w19050, "分辨率"=0.001) -> ("低字节 2"=w19036:dbl, "高字节 2"=w19037:dbl, "低字节"=w19060:dbl, "高字节1"=w19061:dbl)  [unwired: 1 in, 3 out]
                    n7469 = call "输入分辨率计算-EV05.vi"("1字节?"=FALSE, "数值"=w19049, "分辨率"=0.1) -> ("低字节"=w19058:dbl, "高字节1"=w19059:dbl)  [unwired: 2 in, 5 out]
                    n7470 = call "输入分辨率计算-EV05.vi"("1字节?"=TRUE, "数值 2"=w19047, "数值"=w19048, "偏移量"=-40.0, "分辨率"=1.0) -> ("高字节 2"=w19053:dbl, "高字节1"=w19057:dbl)  [unwired: 5 out]
                    n7471 = call "输入分辨率计算-EV05.vi"("1字节?"=FALSE, "数值 2"=w19045, "数值"=w19046, "偏移量"=0.0, "分辨率"=0.1) -> ("低字节 2"=w19042:dbl, "高字节 2"=w19043:dbl, "低字节"=w19055:dbl, "高字节1"=w19056:dbl)  [unwired: 3 out]
                    n7472 = Quotient & Remainder(x=w19041, y=256.0) -> (x-y*floor(x/y)=w19038:dbl, floor(x/y)=w19039:dbl)
                    n7473 = Build Array(w19061, w19060, w19059, w19058, w19057, w19053, w19056, w19055, w19043, w19042, w19039, w19038, w19037, w19036) -> (w19054:dbl[])
                  }
                }
              }
            }
          }
        }
        frame "均衡参数" {
          w19076 = 2
          n7474 = Unbundle By Name(w19079) -> ("均衡参数"=w19074:refnum<vi>)
          n7475 = property class="Clust (严格)"(reference=w19074) -> ("Value"=w19073:T10)  [unwired: 1 in, 2 out]
          n7476 = for {
            N: w19076 -> [_]
            tunnel: [w19087] -> w19081 mode=indexing
            tunnel: [w19086] -> w19080 mode=indexing
            tunnel: w19073 -> [w19085]
            tunnel: [w19084] -> w19078 mode=indexing
            tunnel: [w19082] -> w19075 mode=indexing
            i -> [w19083]
            n7477 = case shown="0, 默认" w19083 {
              tunnel: [24 ("命令序号") 22 ("单个参数补充")] -> w19087
              tunnel: [u32 1 ("命令序号") u32 2 ("命令序号")] -> w19086
              tunnel: w19085 -> [w19118 w19171]
              tunnel: [w19117 w19143] -> w19084
              tunnel: ["均衡阀值" "充电结束电压"] -> w19082
              frame 0, Default {
                n7478 = Unbundle By Name(w19118) -> ("均衡计算-电压高阀值2级"=w19108:sgl, "均衡计算-电压高阀值1级"=w19107:sgl, "均衡计算-电压低阀值1级"=w19106:sgl, "均衡计算-电压低阀值2级"=w19105:sgl, "均衡计算-最低电压阀值"=w19104:sgl, "均衡停止-最低电压阀值"=w19103:sgl, "均衡计算-电压极差阀值"=w19102:sgl)
                n7479 = call "输入分辨率计算-EV05.vi"("1字节?"=FALSE, "数值"=w19102, "分辨率"=0.001) -> ("低字节"=w19088:dbl, "高字节1"=w19089:dbl)  [unwired: 2 in, 5 out]
                n7480 = call "输入分辨率计算-EV05.vi"("1字节?"=FALSE, "数值 2"=w19103, "数值"=w19104, "分辨率"=0.001) -> ("低字节 2"=w19090:dbl, "高字节 2"=w19091:dbl, "低字节"=w19092:dbl, "高字节1"=w19093:dbl)  [unwired: 1 in, 3 out]
                n7481 = call "输入分辨率计算-EV05.vi"("1字节?"=FALSE, "数值 2"=w19107, "数值"=w19108, "分辨率"=0.001) -> ("低字节 2"=w19098:dbl, "高字节 2"=w19099:dbl, "低字节"=w19100:dbl, "高字节1"=w19101:dbl)  [unwired: 1 in, 3 out]
                n7482 = call "输入分辨率计算-EV05.vi"("1字节?"=FALSE, "数值 2"=w19105, "数值"=w19106, "分辨率"=0.001) -> ("低字节 2"=w19094:dbl, "高字节 2"=w19095:dbl, "低字节"=w19096:dbl, "高字节1"=w19097:dbl)  [unwired: 1 in, 3 out]
                n7483 = Build Array(w19101, w19100, w19099, w19098, w19097, w19096, w19095, w19094, w19093, w19092, w19091, w19090, w19089, w19088) -> (w19117:dbl[])
              }
              frame 1 {
                n7484 = Unbundle By Name(w19171) -> ("充电结束电压(90%)"=w19155:sgl, "充电结束电压(91%)"=w19154:sgl, "充电结束电压(92%)"=w19153:sgl, "充电结束电压(93%)"=w19152:sgl, "充电结束电压(94%)"=w19151:sgl, "充电结束电压(95%)"=w19150:sgl, "充电结束电压(96%)"=w19149:sgl, "充电结束电压(97%)"=w19148:sgl, "充电结束电压(98%)"=w19147:sgl, "充电结束电压(99%)"=w19146:sgl, "充电结束电压(100%)"=w19145:sgl)
                n7485 = call "输入分辨率计算-EV05.vi"("1字节?"=FALSE, "数值 2"=w19152, "数值"=w19153, "分辨率"=0.001) -> ("低字节 2"=w19136:dbl, "高字节 2"=w19137:dbl, "低字节"=w19138:dbl, "高字节1"=w19139:dbl)  [unwired: 1 in, 3 out]
                n7486 = call "输入分辨率计算-EV05.vi"("1字节?"=FALSE, "数值 2"=w19150, "数值"=w19151, "分辨率"=0.001) -> ("低字节 2"=w19132:dbl, "高字节 2"=w19133:dbl, "低字节"=w19134:dbl, "高字节1"=w19135:dbl)  [unwired: 1 in, 3 out]
                n7487 = call "输入分辨率计算-EV05.vi"("1字节?"=FALSE, "数值"=w19145, "分辨率"=0.001) -> ("低字节"=w19122:dbl, "高字节1"=w19123:dbl)  [unwired: 2 in, 5 out]
                n7488 = call "输入分辨率计算-EV05.vi"("1字节?"=FALSE, "数值 2"=w19146, "数值"=w19147, "分辨率"=0.001) -> ("低字节 2"=w19124:dbl, "高字节 2"=w19125:dbl, "低字节"=w19126:dbl, "高字节1"=w19127:dbl)  [unwired: 1 in, 3 out]
                n7489 = call "输入分辨率计算-EV05.vi"("1字节?"=FALSE, "数值 2"=w19154, "数值"=w19155, "分辨率"=0.001) -> ("低字节 2"=w19140:dbl, "高字节 2"=w19141:dbl, "低字节"=w19142:dbl, "高字节1"=w19144:dbl)  [unwired: 1 in, 3 out]
                n7490 = call "输入分辨率计算-EV05.vi"("1字节?"=FALSE, "数值 2"=w19148, "数值"=w19149, "分辨率"=0.001) -> ("低字节 2"=w19128:dbl, "高字节 2"=w19129:dbl, "低字节"=w19130:dbl, "高字节1"=w19131:dbl)  [unwired: 1 in, 3 out]
                n7491 = Build Array(w19144, w19142, w19141, w19140, w19139, w19138, w19137, w19136, w19135, w19134, w19133, w19132, w19131, w19130, w19129, w19128, w19127, w19126, w19125, w19124, w19123, w19122) -> (w19143:dbl[])
              }
            }
          }
        }
        frame "均衡阀值" {
          w19175 = 1
          n7492 = Unbundle By Name(w19178) -> ("均衡参数"=w19173:refnum<vi>)
          n7493 = property class="Clust (严格)"(reference=w19173) -> ("Value"=w19172:T10)  [unwired: 1 in, 2 out]
          n7494 = for {
            N: w19175 -> [_]
            tunnel: [w19186] -> w19180 mode=indexing
            tunnel: [w19185] -> w19179 mode=indexing
            tunnel: w19172 -> [w19184]
            tunnel: [w19183] -> w19177 mode=indexing
            tunnel: [w19181] -> w19174 mode=indexing
            i -> [w19182]
            n7495 = case shown="0, 默认" w19182 {
              tunnel: [24 ("命令序号") 22 ("单个参数补充")] -> w19186
              tunnel: [u32 1 ("命令序号") u32 2 ("命令序号")] -> w19185
              tunnel: w19184 -> [w19217 w19270]
              tunnel: [w19216 w19242] -> w19183
              tunnel: ["均衡阀值" "充电结束电压"] -> w19181
              frame 0, Default {
                n7496 = Unbundle By Name(w19217) -> ("均衡计算-电压高阀值2级"=w19207:sgl, "均衡计算-电压高阀值1级"=w19206:sgl, "均衡计算-电压低阀值1级"=w19205:sgl, "均衡计算-电压低阀值2级"=w19204:sgl, "均衡计算-最低电压阀值"=w19203:sgl, "均衡停止-最低电压阀值"=w19202:sgl, "均衡计算-电压极差阀值"=w19201:sgl)
                n7497 = call "输入分辨率计算-EV05.vi"("1字节?"=FALSE, "数值"=w19201, "分辨率"=0.001) -> ("低字节"=w19187:dbl, "高字节1"=w19188:dbl)  [unwired: 2 in, 5 out]
                n7498 = call "输入分辨率计算-EV05.vi"("1字节?"=FALSE, "数值 2"=w19202, "数值"=w19203, "分辨率"=0.001) -> ("低字节 2"=w19189:dbl, "高字节 2"=w19190:dbl, "低字节"=w19191:dbl, "高字节1"=w19192:dbl)  [unwired: 1 in, 3 out]
                n7499 = call "输入分辨率计算-EV05.vi"("1字节?"=FALSE, "数值 2"=w19206, "数值"=w19207, "分辨率"=0.001) -> ("低字节 2"=w19197:dbl, "高字节 2"=w19198:dbl, "低字节"=w19199:dbl, "高字节1"=w19200:dbl)  [unwired: 1 in, 3 out]
                n7500 = call "输入分辨率计算-EV05.vi"("1字节?"=FALSE, "数值 2"=w19204, "数值"=w19205, "分辨率"=0.001) -> ("低字节 2"=w19193:dbl, "高字节 2"=w19194:dbl, "低字节"=w19195:dbl, "高字节1"=w19196:dbl)  [unwired: 1 in, 3 out]
                n7501 = Build Array(w19200, w19199, w19198, w19197, w19196, w19195, w19194, w19193, w19192, w19191, w19190, w19189, w19188, w19187) -> (w19216:dbl[])
              }
              frame 1 {
                n7502 = Unbundle By Name(w19270) -> ("充电结束电压(90%)"=w19254:sgl, "充电结束电压(91%)"=w19253:sgl, "充电结束电压(92%)"=w19252:sgl, "充电结束电压(93%)"=w19251:sgl, "充电结束电压(94%)"=w19250:sgl, "充电结束电压(95%)"=w19249:sgl, "充电结束电压(96%)"=w19248:sgl, "充电结束电压(97%)"=w19247:sgl, "充电结束电压(98%)"=w19246:sgl, "充电结束电压(99%)"=w19245:sgl, "充电结束电压(100%)"=w19244:sgl)
                n7503 = call "输入分辨率计算-EV05.vi"("1字节?"=FALSE, "数值 2"=w19251, "数值"=w19252, "分辨率"=0.001) -> ("低字节 2"=w19235:dbl, "高字节 2"=w19236:dbl, "低字节"=w19237:dbl, "高字节1"=w19238:dbl)  [unwired: 1 in, 3 out]
                n7504 = call "输入分辨率计算-EV05.vi"("1字节?"=FALSE, "数值 2"=w19249, "数值"=w19250, "分辨率"=0.001) -> ("低字节 2"=w19231:dbl, "高字节 2"=w19232:dbl, "低字节"=w19233:dbl, "高字节1"=w19234:dbl)  [unwired: 1 in, 3 out]
                n7505 = call "输入分辨率计算-EV05.vi"("1字节?"=FALSE, "数值"=w19244, "分辨率"=0.001) -> ("低字节"=w19221:dbl, "高字节1"=w19222:dbl)  [unwired: 2 in, 5 out]
                n7506 = call "输入分辨率计算-EV05.vi"("1字节?"=FALSE, "数值 2"=w19245, "数值"=w19246, "分辨率"=0.001) -> ("低字节 2"=w19223:dbl, "高字节 2"=w19224:dbl, "低字节"=w19225:dbl, "高字节1"=w19226:dbl)  [unwired: 1 in, 3 out]
                n7507 = call "输入分辨率计算-EV05.vi"("1字节?"=FALSE, "数值 2"=w19253, "数值"=w19254, "分辨率"=0.001) -> ("低字节 2"=w19239:dbl, "高字节 2"=w19240:dbl, "低字节"=w19241:dbl, "高字节1"=w19243:dbl)  [unwired: 1 in, 3 out]
                n7508 = call "输入分辨率计算-EV05.vi"("1字节?"=FALSE, "数值 2"=w19247, "数值"=w19248, "分辨率"=0.001) -> ("低字节 2"=w19227:dbl, "高字节 2"=w19228:dbl, "低字节"=w19229:dbl, "高字节1"=w19230:dbl)  [unwired: 1 in, 3 out]
                n7509 = Build Array(w19243, w19241, w19240, w19239, w19238, w19237, w19236, w19235, w19234, w19233, w19232, w19231, w19230, w19229, w19228, w19227, w19226, w19225, w19224, w19223, w19222, w19221) -> (w19242:dbl[])
              }
            }
          }
        }
        frame "充电结束电压" {
          w19274 = 1
          n7510 = Unbundle By Name(w19277) -> ("均衡参数"=w19272:refnum<vi>)
          n7511 = property class="Clust (严格)"(reference=w19272) -> ("Value"=w19271:T10)  [unwired: 1 in, 2 out]
          n7512 = for {
            N: w19274 -> [_]
            tunnel: [w19285] -> w19279 mode=indexing
            tunnel: [w19284] -> w19278 mode=indexing
            tunnel: w19271 -> [w19283]
            tunnel: [w19282] -> w19276 mode=indexing
            tunnel: [w19280] -> w19273 mode=indexing
            i -> [w19281]
            n7513 = case shown="0, 默认" w19281 {
              tunnel: [22 ("单个参数补充") 24 ("命令序号")] -> w19285
              tunnel: [u32 2 ("命令序号") u32 1 ("命令序号")] -> w19284
              tunnel: w19283 -> [w19335 w19366]
              tunnel: [w19307 w19365] -> w19282
              tunnel: ["充电结束电压" "均衡阀值"] -> w19280
              frame 0, Default {
                n7514 = Unbundle By Name(w19335) -> ("充电结束电压(90%)"=w19319:sgl, "充电结束电压(91%)"=w19318:sgl, "充电结束电压(92%)"=w19317:sgl, "充电结束电压(93%)"=w19316:sgl, "充电结束电压(94%)"=w19315:sgl, "充电结束电压(95%)"=w19314:sgl, "充电结束电压(96%)"=w19313:sgl, "充电结束电压(97%)"=w19312:sgl, "充电结束电压(98%)"=w19311:sgl, "充电结束电压(99%)"=w19310:sgl, "充电结束电压(100%)"=w19309:sgl)
                n7515 = call "输入分辨率计算-EV05.vi"("1字节?"=FALSE, "数值 2"=w19316, "数值"=w19317, "分辨率"=0.001) -> ("低字节 2"=w19300:dbl, "高字节 2"=w19301:dbl, "低字节"=w19302:dbl, "高字节1"=w19303:dbl)  [unwired: 1 in, 3 out]
                n7516 = call "输入分辨率计算-EV05.vi"("1字节?"=FALSE, "数值 2"=w19314, "数值"=w19315, "分辨率"=0.001) -> ("低字节 2"=w19296:dbl, "高字节 2"=w19297:dbl, "低字节"=w19298:dbl, "高字节1"=w19299:dbl)  [unwired: 1 in, 3 out]
                n7517 = call "输入分辨率计算-EV05.vi"("1字节?"=FALSE, "数值"=w19309, "分辨率"=0.001) -> ("低字节"=w19286:dbl, "高字节1"=w19287:dbl)  [unwired: 2 in, 5 out]
                n7518 = call "输入分辨率计算-EV05.vi"("1字节?"=FALSE, "数值 2"=w19310, "数值"=w19311, "分辨率"=0.001) -> ("低字节 2"=w19288:dbl, "高字节 2"=w19289:dbl, "低字节"=w19290:dbl, "高字节1"=w19291:dbl)  [unwired: 1 in, 3 out]
                n7519 = call "输入分辨率计算-EV05.vi"("1字节?"=FALSE, "数值 2"=w19318, "数值"=w19319, "分辨率"=0.001) -> ("低字节 2"=w19304:dbl, "高字节 2"=w19305:dbl, "低字节"=w19306:dbl, "高字节1"=w19308:dbl)  [unwired: 1 in, 3 out]
                n7520 = call "输入分辨率计算-EV05.vi"("1字节?"=FALSE, "数值 2"=w19312, "数值"=w19313, "分辨率"=0.001) -> ("低字节 2"=w19292:dbl, "高字节 2"=w19293:dbl, "低字节"=w19294:dbl, "高字节1"=w19295:dbl)  [unwired: 1 in, 3 out]
                n7521 = Build Array(w19308, w19306, w19305, w19304, w19303, w19302, w19301, w19300, w19299, w19298, w19297, w19296, w19295, w19294, w19293, w19292, w19291, w19290, w19289, w19288, w19287, w19286) -> (w19307:dbl[])
              }
              frame 1 {
                n7522 = Unbundle By Name(w19366) -> ("均衡计算-电压高阀值1级"=w19356:sgl, "均衡计算-电压高阀值2级"=w19355:sgl, "均衡计算-电压低阀值1级"=w19354:sgl, "均衡计算-电压低阀值2级"=w19353:sgl, "均衡计算-最低电压阀值"=w19352:sgl, "均衡停止-最低电压阀值"=w19351:sgl, "均衡计算-电压极差阀值"=w19350:sgl)
                n7523 = call "输入分辨率计算-EV05.vi"("1字节?"=FALSE, "数值"=w19350, "分辨率"=0.001) -> ("低字节"=w19336:dbl, "高字节1"=w19337:dbl)  [unwired: 2 in, 5 out]
                n7524 = call "输入分辨率计算-EV05.vi"("1字节?"=FALSE, "数值 2"=w19351, "数值"=w19352, "分辨率"=0.001) -> ("低字节 2"=w19338:dbl, "高字节 2"=w19339:dbl, "低字节"=w19340:dbl, "高字节1"=w19341:dbl)  [unwired: 1 in, 3 out]
                n7525 = call "输入分辨率计算-EV05.vi"("1字节?"=FALSE, "数值 2"=w19355, "数值"=w19356, "分辨率"=0.001) -> ("低字节 2"=w19346:dbl, "高字节 2"=w19347:dbl, "低字节"=w19348:dbl, "高字节1"=w19349:dbl)  [unwired: 1 in, 3 out]
                n7526 = call "输入分辨率计算-EV05.vi"("1字节?"=FALSE, "数值 2"=w19353, "数值"=w19354, "分辨率"=0.001) -> ("低字节 2"=w19342:dbl, "高字节 2"=w19343:dbl, "低字节"=w19344:dbl, "高字节1"=w19345:dbl)  [unwired: 1 in, 3 out]
                n7527 = Build Array(w19349, w19348, w19347, w19346, w19345, w19344, w19343, w19342, w19341, w19340, w19339, w19338, w19337, w19336) -> (w19365:dbl[])
              }
            }
          }
        }
        frame "电池包信息1" {
          n7528 = case shown="真" w19373 {
            tunnel: [_ w19386] -> w19377
            tunnel: [_ w19385] -> w19376
            tunnel: w19375 -> [_ w19381]
            tunnel: [_ w19384] -> w19374
            tunnel: [_ u32 35 ("命令序号")] -> w19372
            tunnel: [_ w19379] -> w19371
            tunnel: [_ w19378] -> w19370
            frame False {
            }
            frame True {
              w19379 = 1
              n7529 = Unbundle By Name(w19381) -> ("电池组信息(从板)"=w19382:refnum<vi>)
              n7530 = property class="Clust (严格)"(reference=w19382) -> ("Value"=w19380:T9)  [unwired: 1 in, 2 out]
              n7531 = for {
                N: w19379 -> [_]
                tunnel: [w19392] -> w19386 mode=indexing
                tunnel: [w19391] -> w19385 mode=indexing
                tunnel: w19380 -> [w19390]
                tunnel: [w19389] -> w19384 mode=indexing
                tunnel: [w19387] -> w19378 mode=indexing
                i -> [w19388]
                n7532 = case shown="0, 默认" w19388 {
                  tunnel: [30 ("单个参数补充") 4 ("单个参数补充") 8 ("单个参数补充") 6 ("单个参数补充") 4 ("单个参数补充") 8 ("单个参数补充") 14 ("单个参数补充")] -> w19392
                  tunnel: [u32 1 ("命令序号") u32 2 ("命令序号") u32 3 ("命令序号") u32 4 ("命令序号") u32 5 ("命令序号") u32 6 ("命令序号") u32 7 ("命令序号")] -> w19391
                  tunnel: w19390 -> [w19396 w19471 w19479 w19509 w19520 w19528 w19549]
                  tunnel: [w19393 w19464 w19496 w19511 w19521 w19526 w19551] -> w19389
                  tunnel: ["电池包信息1" "电池包序号" "充放电安时" "充电次数时间" "SOC" "车牌号" "充电参数"] -> w19387
                  frame 0, Default {
                    w19406 = ":" ("正则表达式")
                    w19414 = 0.0 ("元素")
                    w19433 = 256.0 ("y")
                    w19438 = 256.0 ("y")
                    w19451 = 2 ("偏移量(0)")
                    w19448 = "-" ("正则表达式")
                    # "电池组信息"
                    n7533 = Unbundle By Name(w19396) -> ("串联数"=w19455:dbl, "并联数"=w19454:dbl, "电池厂家"=w19394:dbl, "电池类型"=w19395:dbl, "生产日期"=w19453:string)
                    n7534 = Unbundle By Name(w19396) -> ("额定能量"=w19419:dbl, "额定容量"=w19421:dbl, "实际容量"=w19420:dbl, "额定总压"=w19444:dbl)
                    n7535 = Match Pattern(string=w19453, regular expression=w19448) -> (before substring=w19452:string, after substring=w19449:string)  [unwired: 3 out]
                    n7536 = Match Pattern(string=w19449, regular expression=w19448) -> (before substring=w19447:string, after substring=w19412:string)  [unwired: 3 out]
                    n7537 = Match Pattern(string=w19412, regular expression=" " ("正则表达式")) -> (before substring=w19410:string, after substring=w19409:string)  [unwired: 3 out]
                    n7538 = call "输入分辨率计算-EV05.vi"("1字节?"=FALSE, "数值"=w19419, "分辨率"=0.1) -> ("低字节"=w19418:dbl, "高字节1"=w19417:dbl)  [unwired: 2 in, 5 out]
                    n7539 = String Subset(string=w19452, offset (0)=w19451, length (rest)=w19451) -> (substring=w19450:string)
                    n7540 = call "输入分辨率计算-EV05.vi"("1字节?"=TRUE, "数值 2"=w19420, "数值"=w19421, "分辨率"=0.001) -> ("高字节 2"=w19422:dbl, "高字节1"=w19423:dbl)  [unwired: 1 in, 5 out]
                    n7541 = Match Pattern(string=w19409, regular expression=w19406) -> (before substring=w19408:string, after substring=w19407:string)  [unwired: 3 out]
                    n7542 = Fract/Exp String To Number(string=w19450) -> (number=w19402:dbl)  [unwired: 1 in, 3 out]
                    n7543 = Fract/Exp String To Number(string=w19447) -> (number=w19401:dbl)  [unwired: 4 out]
                    n7544 = Fract/Exp String To Number(string=w19410) -> (number=w19400:dbl)  [unwired: 4 out]
                    n7545 = Match Pattern(string=w19407, regular expression=w19406) -> (before substring=w19405:string, after substring=w19404:string)  [unwired: 3 out]
                    n7546 = call "输入分辨率计算-EV05.vi"("1字节?"=FALSE, "数值"=w19444, "分辨率"=0.1) -> ("低字节"=w19415:dbl, "高字节1"=w19416:dbl)  [unwired: 2 in, 5 out]
                    n7547 = Quotient & Remainder(x=w19423, y=w19438) -> (x-y*floor(x/y)=w19437:dbl, floor(x/y)=w19441:dbl)
                    n7548 = Fract/Exp String To Number(string=w19408) -> (number=w19399:dbl)  [unwired: 4 out]
                    n7549 = Quotient & Remainder(x=w19422, y=w19433) -> (x-y*floor(x/y)=w19429:dbl, floor(x/y)=w19430:dbl)
                    n7550 = Quotient & Remainder(x=w19441, y=w19438) -> (x-y*floor(x/y)=w19436:dbl, floor(x/y)=w19440:dbl)
                    n7551 = Fract/Exp String To Number(string=w19405) -> (number=w19398:dbl)  [unwired: 4 out]
                    n7552 = Quotient & Remainder(x=w19430, y=w19433) -> (x-y*floor(x/y)=w19428:dbl, floor(x/y)=w19431:dbl)
                    n7553 = call <vilib>:"Trim Whitespace.vi"("string"=w19404) -> ("trimmed string"=w19403:string)  [unwired: 1 in]
                    n7554 = Quotient & Remainder(x=w19440, y=w19438) -> (x-y*floor(x/y)=w19435:dbl, floor(x/y)=w19439:dbl)
                    n7555 = Quotient & Remainder(x=w19431, y=w19433) -> (x-y*floor(x/y)=w19427:dbl, floor(x/y)=w19432:dbl)
                    n7556 = Quotient & Remainder(x=w19455, y=256.0) -> (x-y*floor(x/y)=w19457:dbl, floor(x/y)=w19458:dbl)
                    n7557 = Fract/Exp String To Number(string=w19403) -> (number=w19397:dbl)  [unwired: 4 out]
                    n7558 = Quotient & Remainder(x=w19439, y=w19438) -> (x-y*floor(x/y)=w19434:dbl)  [unwired: 1 out]
                    n7559 = Quotient & Remainder(x=w19432, y=w19433) -> (x-y*floor(x/y)=w19426:dbl)  [unwired: 1 out]
                    n7560 = Build Array(w19417, w19418, w19434, w19435, w19436, w19437, w19426, w19427, w19428, w19429, w19416, w19415, w19414, w19414, w19414, w19402, w19401, w19400, w19399, w19398, w19397) -> (w19413:dbl[])
                    n7561 = Build Array(w19458, w19457, w19454, w19394, w19395) -> (w19456:dbl[])
                    n7562 = Insert Into Array(array=w19456, new element=w19413) -> (w19393:dbl[])  [unwired: 1 in]
                  }
                  frame 1 {
                    n7563 = Unbundle By Name(w19471) -> ("电池包序号"=w19468:dbl)
                    n7564 = Quotient & Remainder(x=w19468, y=256.0) -> (x-y*floor(x/y)=w19465:dbl, floor(x/y)=w19466:dbl)
                    n7565 = Build Array(w19466, w19465) -> (w19464:dbl[])
                  }
                  frame 2 {
                    w19487 = 256.0 ("y")
                    w19492 = 256.0 ("y")
                    # "充放电安时/安时数"
                    n7566 = Unbundle By Name(w19479) -> ("充电总安时"=w19476:dbl, "放电总这时"=w19475:dbl)
                    n7567 = call "输入分辨率计算-EV05.vi"("1字节?"=TRUE, "数值 2"=w19475, "数值"=w19476, "分辨率"=0.001) -> ("高字节 2"=w19473:dbl, "高字节1"=w19474:dbl)  [unwired: 1 in, 5 out]
